vi "SET - Triggered Events & Data.vi"(8 "error in (no error)":errorcluster, 9 "Data":string="Hi!!!", 10 "Events":T1, 11 "Child_6_Class in":refnum<class "Embedded_DB_Class.lvclass">) -> (0 "error out":errorcluster, 3 "Child_6_Class out":refnum<class "Embedded_DB_Class.lvclass">)   [LabVIEW 2023, in "Embedded_DB_Actor.lvlib" / "Embedded_DB_Class.lvclass"]
uses:
  Embedded_DB_Class.lvclass
  Abstraction_Interface_Class/Usr Ev/Ctrl - Enum - Events.ctl
  Abstraction_Interface_Class/Abstraction_Interface_Class.lvclass
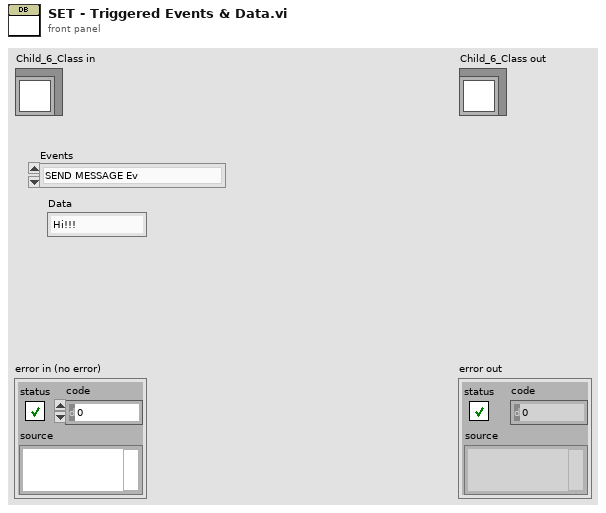
[diagram p1: front panel]
types:
  T1 = typedef "Abstraction_Interface.lvlib/Abstraction_Interface_Class.lvclass/Ctrl - Enum - Events.ctl" = enum16{"SEND MESSAGE Ev", "STOP_ACTOR Ev", "INIT_ACTOR Ev", "START Ev", "STOP Ev", "GET Ev", "SET Ev", "ERROR_HANDLER Ev", "RESET Ev"}
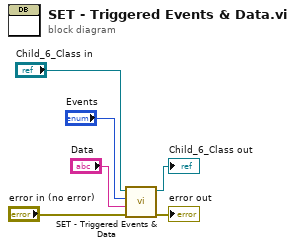
[diagram p0: block diagram]
diagram:
  n1 = call-parent "SET - Triggered Events & Data.vi"("error in (no error)"="error in (no error)", "Data"="Data", "Events"="Events", "Interface_Class in"="Child_6_Class in") -> ("error out"=→"error out":errorcluster, "Interface_Class out"=→"Child_6_Class out":refnum<class "Embedded_DB_Class.lvclass">)  [unwired: 6 in]
